vi "Do.vi"(8 "error in (no error)":errorcluster, 10 "Actor in":refnum<class "Actor.lvclass">, 11 "ConfigureAppenderMsg":refnum<class "ConfigureAppenderMsg.lvclass">) -> (0 "error out":errorcluster, 2 "Actor out":refnum<class "Actor.lvclass">)   [LabVIEW 2026, in "Lumberjack.lvlib" / "ConfigureAppenderMsg.lvclass"]
doc: "<p>(<strong>Filename</strong>: <span class=\"dnl\">Actor Framework.lvlib:Message.lvclass:Do.vi</span>)</p>\n<p>Defines what a message does when it is received by an actor. Generally, a message instructs an actor to invoke one of its methods. By default, this method does nothing. A child class must override it to define behavior.</p>"
uses:
  ConfigureAppenderMsg.lvclass
  <vilib>/ActorFramework/Actor/Actor.lvclass
  LogManager/LogManager.lvclass/LogManager.lvclass
  C:/Program Files (x86)/National Instruments/LabVIEW 2026/vi.lib/ActorFramework/Actor/Actor.lvclass
  ConfigureAppenderMsg.lvclass/ConfigureAppenderMsg.ctl
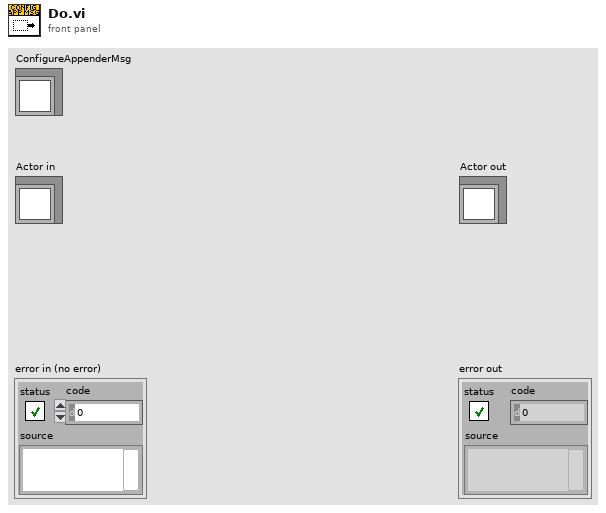
[diagram p1: front panel]
types:
  T1 = typedef "Lumberjack.lvlib/Filter.ctl" = cluster{"mode":T2, "levelMin":T3, "levelMax":T3, "tagPrefix":string}
  T2 = typedef "Lumberjack.lvlib/FilterMode.ctl" = enum16{"Mirror", "Routed"}
  T3 = typedef "Lumberjack.lvlib/Severity.ctl" = enum16{"OFF", "FATAL", "ERROR", "WARN", "INFO", "DEBUG", "TRACE", "ALL"}
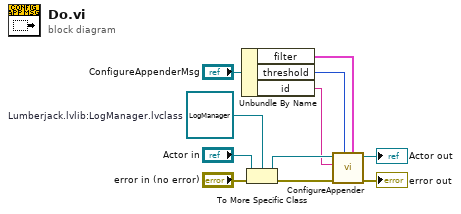
[diagram p0: block diagram]
diagram:
  w9 = refnum<class "LogManager.lvclass"> refnum  # Lumberjack.lvlib:LogManager.lvclass
  n1 = Unbundle By Name("ConfigureAppenderMsg") -> ("filter"=w3:T1, "threshold"=w2:T3, "id"=w1:string)
  n2 = To More Specific Class(target class=w9, reference="Actor in", error in="error in (no error)") -> (specific class reference=w7:refnum<class "LogManager.lvclass">, error out=w8:errorcluster)
  n3 = call "ConfigureAppender.vi"("filter"=w3, "threshold"=w2, "error in (no error)"=w8, "id"=w1, "LogManager in"=w7) -> ("error out"=→"error out":errorcluster, "LogManager out"=→"Actor out":refnum<class "LogManager.lvclass">)  [unwired: 5 in]
